vi "ETH2_E1A_Offset.vi"(0 "RTD1 Offset 1":dbl, 1 "RTD2 Offset":dbl, 2 "RTD3 Offset":dbl, 3 "RTD4 Offset":dbl, 4 "RTD5 Offset":dbl, 5 "RTD6 Offset":dbl, 6 "Write/Read":enum16{"Write", "Read"}(ring)=enum."Read") -> (14 "RTD1 Offset Out":dbl, 15 "RTD2 Offset Out":dbl, 16 "RTD3 Offset Out":dbl, 17 "RTD4 Offset out":dbl, 18 "RTD5 Offset out":dbl, 19 "RTD6 Offset  out":dbl)   [LabVIEW 2022 SP3]
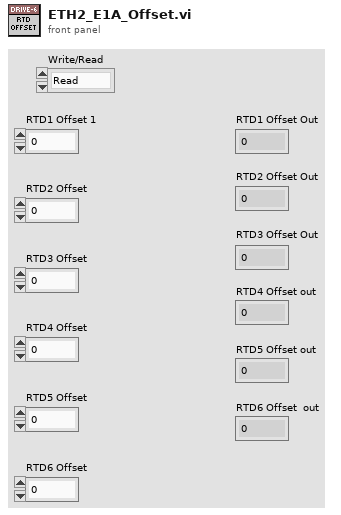
[diagram p1: front panel]
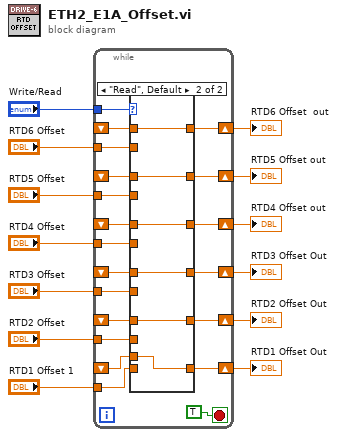
[diagram p0: block diagram]
diagram:
  n1 = while {
    shift-right: [w32] -> w11
    shift-left: _ -> [w30]
    tunnel: "Write/Read" -> [w33]
    tunnel: "RTD1 Offset 1" -> [w31]
    tunnel: "RTD2 Offset" -> [w28]
    shift-right: [w27] -> w9
    shift-left: _ -> [w26]
    tunnel: "RTD3 Offset" -> [w25]
    shift-right: [w24] -> w7
    shift-left: _ -> [w23]
    tunnel: "RTD4 Offset" -> [w22]
    tunnel: "RTD5 Offset" -> [w21]
    tunnel: "RTD6 Offset" -> [w20]
    shift-right: [w19] -> w3
    shift-left: _ -> [w16]
    shift-right: [w18] -> w2
    shift-left: _ -> [w15]
    shift-right: [w17] -> w1
    shift-left: _ -> [w14]
    stop <- TRUE stop-if-true
    n2 = case shown="\"Read\", Default" w33 {
      tunnel: w31 -> [w39 _]
      tunnel: [w39 w45] -> w32
      tunnel: w30 -> [_ w45]
      tunnel: w28 -> [w38 _]
      tunnel: [w38 w44] -> w27
      tunnel: w26 -> [_ w44]
      tunnel: w25 -> [w37 _]
      tunnel: [w37 w43] -> w24
      tunnel: w23 -> [_ w43]
      tunnel: w22 -> [w36 _]
      tunnel: w21 -> [w35 _]
      tunnel: w20 -> [w34 _]
      tunnel: [w36 w42] -> w19
      tunnel: [w35 w41] -> w18
      tunnel: [w34 w40] -> w17
      tunnel: w16 -> [_ w42]
      tunnel: w15 -> [_ w41]
      tunnel: w14 -> [_ w40]
      frame "Write" {
      }
      frame "Read", Default {
      }
    }
  }
  "RTD1 Offset Out" <- w11
  "RTD2 Offset Out" <- w9
  "RTD3 Offset Out" <- w7
  "RTD4 Offset out" <- w3
  "RTD5 Offset out" <- w2
  "RTD6 Offset  out" <- w1
